vi "Step 4 - Model and Simulate FXP Lowpass (Lowpass).vi"() -> ()   [LabVIEW 2023]
doc: "Demonstrates how to use the DFD FXP Modeling VI to model a fixed-point filter, the DFD FXP Simulation VI to simulate the filtering process, the DFD FXP Simulation Report VI to get the statistics of the simulation process, and the DFD Filtering VI to get the reference floating-point filtering results.\n\nThis example uses the DFD FXP Modeling VI to create a model of the fixed-point lowpass filter. The example then uses the DFD FXP Simulation VI to apply the fixed-point lowpass filter model to a signal from the Uniform White Noise VI and simulates the filtering result. This example also uses the DFD FXP Simulation Report VI to generate the statistics of the simulation process. To verify the simulation, this example uses the DFD Filtering VI to filter the same signal that Uniform White Noise VI generates with the reference floating-point lowpass filter and finally compares the filtered signal with the simulation result.\n\nAfter you run this VI, observe the <B>Filtering Text Report</B> output on the front panel. You can use this data to optimize the fixed-point model. For example, you might verify that <B>#Overflows</B> and <B>#Underflows</B> equal 0. You also can compare the signal from the reference floating-point lowpass filter and the signal from the fixed-point lowpass filter model. The ideal result is that the two signals overlap each other."
uses:
  <vilib>/addons/Digital Filter Design/_Objects.llb/DFD Coef Norm Type.ctl
  <vilib>/addons/Digital Filter Design/FXPModel.llb/DFD FXP Quantize Coef (Easy).vi
  <vilib>/addons/Digital Filter Design/Process.llb/DFD Filtering (Array).vi
  <vilib>/Utility/VariantDataType/GetNumericFxpInfo.vi
  <vilib>/addons/Digital Filter Design/FXPSim.llb/dfd_Check Input FXP Settings.vi
  <vilib>/addons/Digital Filter Design/FXPSim.llb/dfd_Check SRate Simulation Integer Input.vi
  <vilib>/addons/Digital Filter Design/FXPSim.llb/dfd_FXP Simu.vi
  <vilib>/addons/Digital Filter Design/_Objects.llb/DFD Quantization Sources.ctl
  <vilib>/addons/Digital Filter Design/_Objects.llb/DFD FXP Statistics Data.ctl
  <vilib>/addons/Digital Filter Design/FXPSim.llb/SimXnode/DFD FXP Simulation.xnode
  <vilib>/addons/Digital Filter Design/_Objects.llb/DFD Filter Obj.ctl
  <vilib>/addons/Digital Filter Design/_Objects.llb/DFD Filter Coef.ctl
  <vilib>/addons/Digital Filter Design/_Objects.llb/DFD Filter Structure Type Selector.ctl
  <vilib>/addons/Digital Filter Design/_Objects.llb/dfd_Internal Quantization Settings.ctl
  <vilib>/addons/Digital Filter Design/_Objects.llb/dfd_Internal Quantization Srcs.ctl
  <vilib>/addons/Digital Filter Design/NI_DigFilterLicensed.lvlib
  <vilib>/addons/Digital Filter Design/NI_DigFilter_FXP.lvlib
  <vilib>/Utility/VariantDataType/VariantType.lvlib
  <vilib>/Analysis/NI_AALBase.lvlib
panel:
  out "Filtered Signals":dbl[][](graph)
  out "Filtering Text Report":string
  # "Select Help>>Show Context Help and move the cursor over the VI icon for more information."
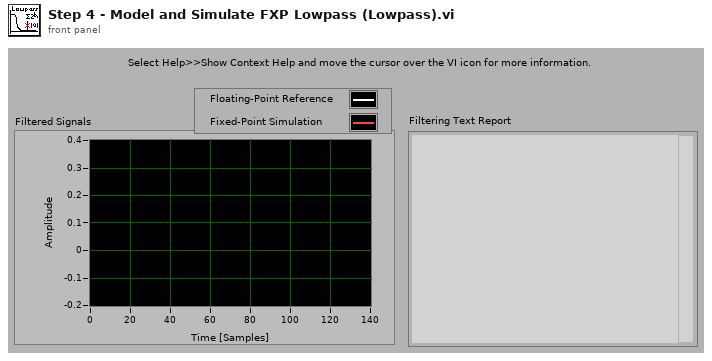
[diagram p1: front panel]
types:
  T1 = typedef "NI_DigFilterLicensed.lvlib/DFD Coef Norm Type.ctl" = enum16{"No Norm", "Time Domain 1-Norm", "Time Domain 2-Norm", "Time Domain Inf-Norm"}
  T2 = typedef "NI_DigFilterLicensed.lvlib/DFD Filter Obj.ctl" = cluster{"mSRate_Fs":dbl, "mSRate_Version":string, "mSRate_Comments":string, "mSRate_OrgCoef":T3, "mSRate_CurCoef":T3, "mSRate_Quantized?":bool, "mSRate_QCoef":T3, "mSRate_QSettings":T5[], "mSRate_Order":i32, "mSRate_Scaling":cluster{"mSRate_ScaleByPowerOf2?":bool, "mSRate_ScaleType":T1}}
  T3 = typedef "NI_DigFilterLicensed.lvlib/DFD Filter Coef.ctl" = cluster{"type":T4, "gain":dbl, "coef a (k)":dbl[], "coef b (v)":dbl[]}
  T4 = typedef "NI_DigFilterLicensed.lvlib/DFD Filter Structure Type Selector.ctl" = enum16{"Undefined", "FIR Direct Form", "FIR Direct Form Transposed", "FIR Symmetric", "FIR Antisymmetric", "IIR Direct Form I", "IIR Direct Form I Transposed", "IIR Direct Form II", "IIR Direct Form II Transposed", "IIR Cascaded Second Order Sections Form I", "IIR Cascaded Second Order Sections Form I Transposed", "IIR Cascaded Second Order Sections Form II", "IIR Cascaded Second Order Sections Form II Transposed", "Lattice Allpass (basic sections)", "Lattice Allpass (one multiplier sections)", "Lattice Allpass (normalized sections)", "Lattice AR (basic sections)", "Lattice AR (one multiplier sections)", "Lattice AR (normalized sections)", "Lattice MA (minimum phase)", "Lattice MA (maximum phase)", "Lattice ARMA (basic sections)", "Lattice ARMA (one multiplier sections)", "Lattice ARMA (normalized sections)"}
  T5 = typedef "NI_DigFilterLicensed.lvlib/dfd_Internal Quantization Settings.ctl" = cluster{"source":T6, "wl":i16, "iwl":i16, "overflow mode":enum16{"Saturation", "Wrap"}, "rounding mode":enum16{"Nearest", "Truncation"}, "signed?":bool}
  T6 = typedef "NI_DigFilterLicensed.lvlib/dfd_Internal Quantization Srcs.ctl" = u16
  T7 = typedef "NI_DigFilterLicensed.lvlib/DFD Quantization Sources.ctl" = u16
  T8 = typedef "NI_DigFilterLicensed.lvlib/DFD FXP Statistics Data.ctl" = cluster{"max value":ext, "min value":ext, "#overflows":i32, "#underflows":i32, "#operations":i32}
  T9 = cluster{"quantizer source":T7, "statistics information":T8}[]
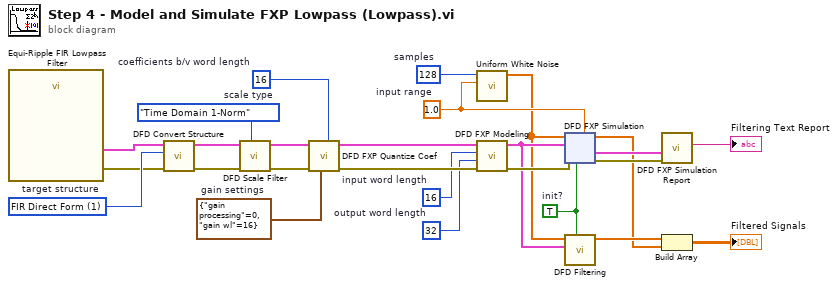
[diagram p0: block diagram]
diagram:
  w3 = i16 32  # output word length
  w4 = i16 16  # input word length
  w16 = i16 16  # coefficients b/v word length
  w26 = u16 1 items=["FIR Direct Form"=1, "FIR Direct Form Transposed"=2, "FIR Symmetric"=3, "FIR Antisymmetric"=4, "IIR Direct Form I"=5, "IIR Direct Form I Transposed"=6, "IIR Direct Form II"=7, "IIR Direct Form II Transposed"=8, "IIR Cascaded Second-Order Sections Form I"=9, "IIR Cascaded Second-Order Sections Form I Transposed"=10, "IIR Cascaded Second-Order Sections Form II"=11, "IIR Cascaded Second-Order Sections Form II Transposed"=12, "Lattice Allpass (basic sections)"=13, "Lattice Allpass (one multiplier sections)"=14, "Lattice Allpass (normalized sections)"=15, "Lattice AR (basic sections)"=16, "Lattice AR (one multiplier sections)"=17, "Lattice AR (normalized sections)"=18, "Lattice MA (minimum phase)"=19, "Lattice MA (maximum phase)"=20, "Lattice ARMA (basic sections)"=21, "Lattice ARMA (one multiplier sections)"=22, "Lattice ARMA (normalized sections)"=23]  # target structure
  w8 = DFD_Coef_Norm_Type."Time Domain 1-Norm"  # scale type
  w13 = cluster{"gain processing":u16, "gain wl":i16} {"gain processing"=0, "gain wl"=16}  # gain settings
  w15 = 1.0  # input range
  w14 = TRUE  # init?
  w25 = 128  # samples
  n1 = call "Equi-Ripple FIR Lowpass Filter"() -> ("error out"=w1:errorcluster, "filter out"=w2:T2)  [unwired: 1 in, 9 out]
  n2 = call <vilib>:"DFD Convert Structure.vi"("error in (no error)"=w1, "target structure"=w26, "filter in"=w2) -> ("error out"=w11:errorcluster, "filter out"=w12:T2)  [unwired: 7 out]
  n3 = call <vilib>:"DFD Scale Filter.vi"("scale type"=w8, "error in (no error)"=w11, "filter in"=w12) -> ("error out"=w10:errorcluster, "filter out"=w9:T2)  [unwired: 7 out]
  n4 = call-poly <vilib>:"DFD FXP Quantize Coef.vi"("coefficients b/v word length"=w16, "gain settings"=w13, "error in (no error)"=w10, "filter in"=w9) -> ("error out"=w17:errorcluster, "filter out"=w18:T2)  [unwired: 1 in, 5 out]
  n5 = call <vilib>:"Uniform White Noise.vi"("amplitude"=w15, "samples"=w25) -> ("uniform white noise"=w5:dbl[])  [unwired: 8 in, 1 out]
  n6 = call <vilib>:"DFD FXP Modeling.vi"("error in (no error)"=w17, "output word length"=w3, "input word length"=w4, "filter in"=w18) -> ("error out"=w7:errorcluster, "filter out"=w6:T2)  [unwired: 3 in, 3 out]
  n7 = xnode "DFD FXP Simulation"("input range"=w15, "init? (T)"=w14, "error in (no error)"=w7, "filter in"=w6, "signal in"=w5) -> ("error out"=w24:errorcluster, "filtering statistics report"=w23:T9, "DBL signal out"=w19:dbl[])  [unwired: 1 in, 1 out]
  n8 = call-poly <vilib>:"DFD Filtering.vi"("init? (F)"=w14, "filter"=w6, "signal in"=w5) -> ("signal out"=w20:dbl[])  [unwired: 1 in, 7 out]
  n9 = call <vilib>:"DFD FXP Simulation Report.vi"("error in (no error)"=w24, "filtering statistics report"=w23) -> ("filtering text report"=→"Filtering Text Report":string)  [unwired: 9 out]
  n10 = Build Array(w20, w19) -> (→"Filtered Signals":dbl[][])
